vi "odor temporal control panel with logging no AO1 on air and odor1.vi"() -> ()   [LabVIEW 2021]
uses:
  Image Aquisition - Labview/Image Recorder/experiment state global.vi
  <vilib>/DAQmx/write.llb/DAQmx Write (Digital Bool 1Line 1Point).vi
panel:
  in  "direct control of digital lines":bool
  in  "digital controls":T1
  out "flow rates":T2
  out "setpoints":T3={"Air "=1.0, "odor1"=0.0, "odor2"=0.0, "co2"=0.0}
  in  "gradient settings":T4={"air settings"={"enabled"=TRUE, "temporal ramp type"=enum."Square", "period(s)"=1200.0, "high limit"=4.0, "low limit"=4.0, "duty cycle (sq wave)"=50.0, "phase shift (deg)"=0.0, "value to output when disabled"=1.0}, "odor1 settings"={"enabled"=FALSE, "temporal ramp type"=enum."Sine", "period(s)"=120.0, "high limit"=0.0, "low limit"=0.0, "duty cycle (sq wave)"=50.0, "phase shift (deg)"=0.0, "value to output when disabled"=0.0}, "odor2 settings"={"enabled"=FALSE, "temporal ramp type"=enum."Sine", "period(s)"=120.0, "high limit"=0.0, "low limit"=0.0, "duty cycle (sq wave)"=50.0, "phase shift (deg)"=0.0, "value to output when disabled"=0.0}, "co2 settings"={"enabled"=TRUE, "temporal ramp type"=enum."Triangle", "period(s)"=30.0, "high limit"=500.0, "low limit"=0.0, "duty cycle (sq wave)"=50.0, "phase shift (deg)"=-90.0, "value to output when disabled"=0.0}} {"co2 settings"."value to output when disabled" min=0.0; "co2 settings"."low limit" format="%#_6p"; "odor2 settings"."value to output when disabled" max=100.0; "odor2 settings"."low limit" format="%#_6p"; "odor2 settings"."high limit" max=100.0; "odor1 settings"."value to output when disabled" max=100.0; "odor1 settings"."low limit" format="%#_6p"; "odor1 settings"."high limit" max=100.0; "air settings"."value to output when disabled" max=100.0; "air settings"."low limit" format="%#_6p"; "air settings"."high limit" max=100.0}
  in  "Sync Gradient To Image Aquisition":bool
  in  "enable gradient":bool
  in  "restart gradient":bool
  in  "update period (ms)":u32=100
  in  "stop":bool
  out "error out":errorcluster
  # "restarting gradient also enables output"
  # "maximum amplitude is 100"
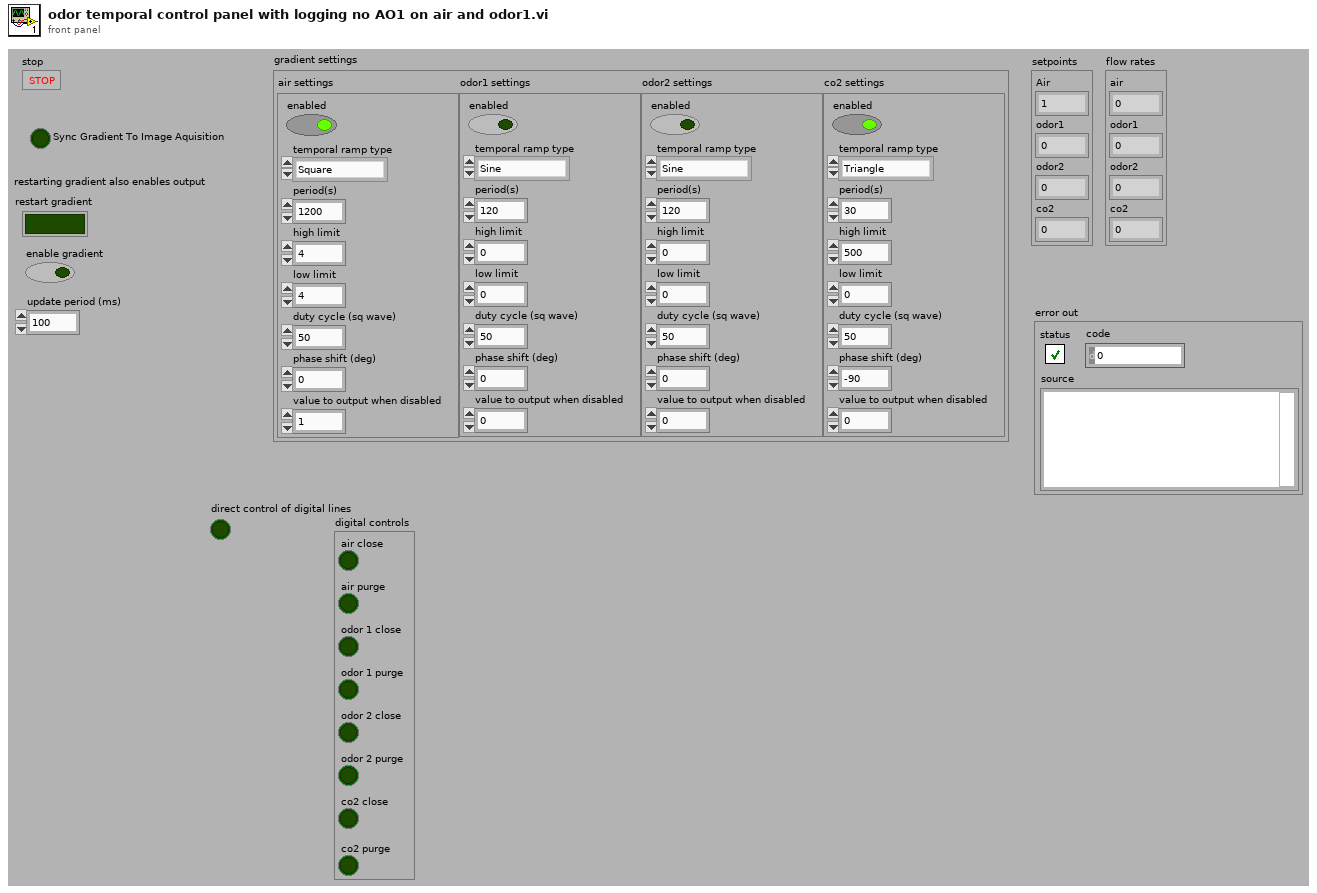
[diagram p1: front panel]
types:
  T1 = cluster{"air close":bool, "air purge":bool, "odor 1 close":bool, "odor 1 purge":bool, "odor 2 close":bool, "odor 2 purge":bool, "co2 close":bool, "co2 purge":bool}
  T2 = cluster{"air":dbl, "odor1":dbl, "odor2":dbl, "co2":dbl}
  T3 = cluster{"Air ":dbl, "odor1":dbl, "odor2":dbl, "co2":dbl}
  T4 = cluster{"air settings":cluster{"enabled":bool, "temporal ramp type":enum16{"Sine", "Triangle", "Sawtooth", "Square", "Exponential"}, "period(s)":dbl, "high limit":dbl, "low limit":dbl, "duty cycle (sq wave)":dbl, "phase shift (deg)":dbl, "value to output when disabled":dbl}, "odor1 settings":cluster{"enabled":bool, "temporal ramp type":enum16{"Sine", "Triangle", "Sawtooth", "Square", "Exponential"}, "period(s)":dbl, "high limit":dbl, "low limit":dbl, "duty cycle (sq wave)":dbl, "phase shift (deg)":dbl, "value to output when disabled":dbl}, "odor2 settings":cluster{"enabled":bool, "temporal ramp type":enum16{"Sine", "Triangle", "Sawtooth", "Square", "Exponential"}, "period(s)":dbl, "high limit":dbl, "low limit":dbl, "duty cycle (sq wave)":dbl, "phase shift (deg)":dbl, "value to output when disabled":dbl}, "co2 settings":cluster{"enabled":bool, "temporal ramp type":enum16{"Sine", "Triangle", "Sawtooth", "Square", "Exponential"}, "period(s)":dbl, "high limit":dbl, "low limit":dbl, "duty cycle (sq wave)":dbl, "phase shift (deg)":dbl, "value to output when disabled":dbl}}
  T5 = cluster{"analog output channels":cluster{"air ao":refnum<k21>, "odor 1 ao":refnum<k21>, "odor 2 ao":refnum<k21>, "co2 ao":refnum<k21>}, "analog input channels":cluster{"air ai":refnum<k21>, "odor 1 ai":refnum<k21>, "odor 2 ai":refnum<k21>, "co2 ai":refnum<k21>, "pid sensor 1 ai":refnum<k21>, "pid sensor 2 ai":refnum<k21>}, "digital control lines":cluster{"air close":refnum<k21>, "air purge":refnum<k21>, "odor 1 close":refnum<k21>, "odor 1 purge":refnum<k21>, "odor 2 close":refnum<k21>, "odor 2 purge":refnum<k21>, "co2 close":refnum<k21>, "co2 purge":refnum<k21>}}
  T6 = cluster{"experiment started":bool, "experiment ended":bool, "experiment start time":u32}
  T7 = cluster{"air close":refnum<k21>, "air purge":refnum<k21>, "odor 1 close":refnum<k21>, "odor 1 purge":refnum<k21>, "odor 2 close":refnum<k21>, "odor 2 purge":refnum<k21>, "co2 close":refnum<k21>, "co2 purge":refnum<k21>}
  T8 = cluster{"air":dbl, "odor1":dbl, "odor2":dbl, "co2":dbl, "pid reading":dbl}
  T9 = cluster{"data directory":path, "file stub":string}
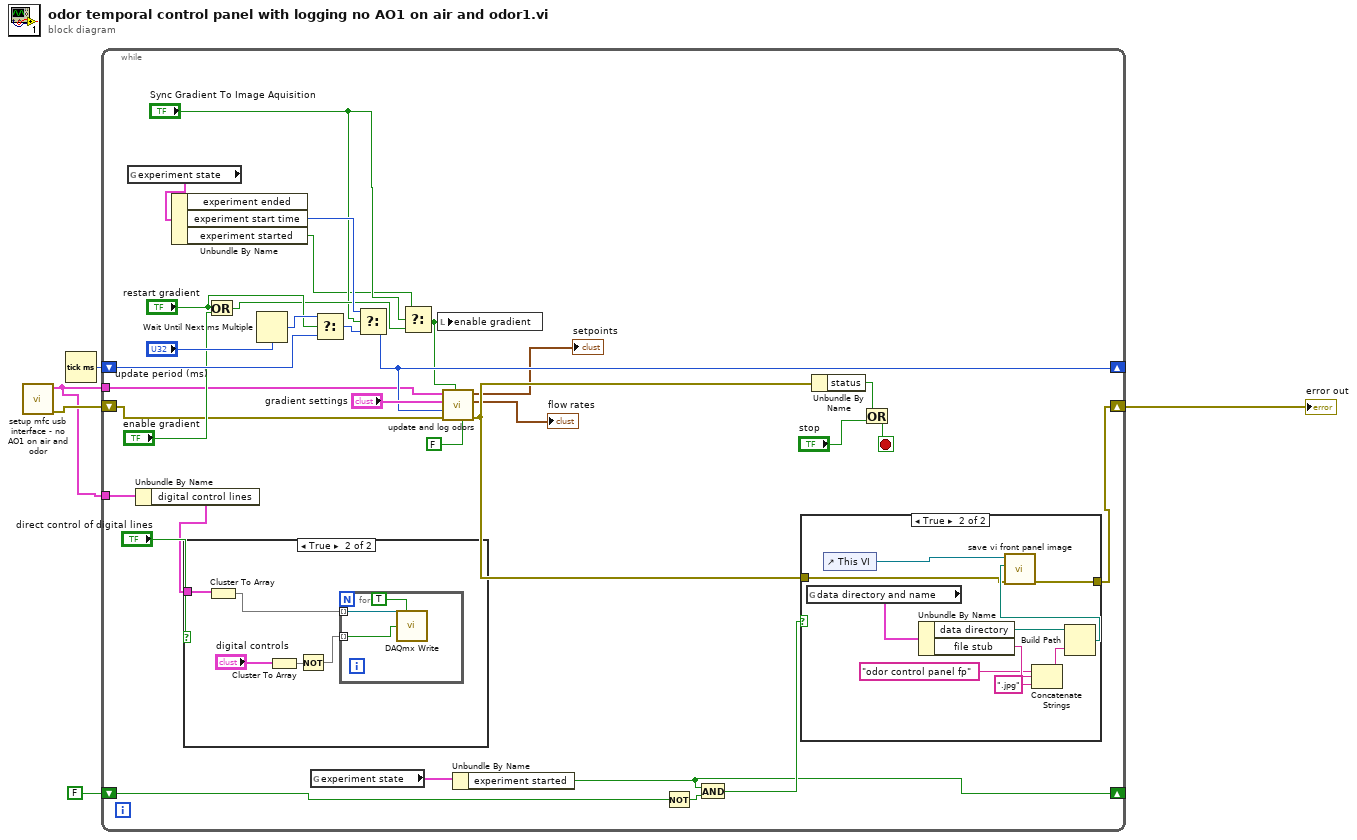
[diagram p0: block diagram]
diagram:
  n1 = call "setup mfc usb interface - no AO1 on air and odor.vi"() -> ("error out"=w4:errorcluster, "daqmx tasks"=w1:T5)  [unwired: 10 in]
  n2 = Tick Count (ms)() -> (millisecond timer value=w5:u32)
  n3 = while {
    shift-right: [w18] -> w3
    shift-left: w4 -> [w15]
    shift-right: [w16] -> _
    shift-left: w5 -> [w34]
    tunnel: w1 -> [w13]
    shift-right: [w20] -> _
    shift-left: FALSE ("experiment started") -> [w19]
    tunnel: w1 -> [w9]
    stop <- w37 stop-if-true
    n4 = global read "experiment state global.vi" "experiment state"() -> (w29:T6)
    n5 = Unbundle By Name(w9) -> ("digital control lines"=w7:T7)
    n6 = Unbundle By Name(w29) -> ("experiment start time"=w28:u32, "experiment started"=w24:bool)  [unwired: 1 out]
    n7 = case shown="True" "direct control of digital lines" {
      tunnel: w7 -> [_ w41]
      frame False {
      }
      frame True {
        n8 = Cluster To Array(cluster=w41) -> (array=w39:refnum<k21>[])
        n9 = Cluster To Array(cluster="digital controls") -> (array=w40:bool[])
        n10 = Not(x=w40) -> (.not. x?=w38:bool[])
        n11 = for {
          tunnel: w39 -> [w45] mode=indexing
          tunnel: w38 -> [w44] mode=indexing
          n12 = call-poly <vilib>:"DAQmx Write.vi"("task/channels in"=w45, "auto start"=TRUE, "data"=w44) -> ()  [unwired: 10 in, 3 out]
        }
      }
    }
    n13 = Or(x="restart gradient", y="enable gradient") -> (x .or. y?=w27:bool)
    n14 = Wait Until Next ms Multiple(millisecond multiple="update period (ms)") -> (millisecond timer value=w33:u32)
    n15 = global read "experiment state global.vi" "experiment state"() -> (w21:T6)
    n16 = Select(t=w33, s="restart gradient", f=w34) -> (s? t:f=w30:u32)
    n17 = Select(t=w28, s="Sync Gradient To Image Aquisition", f=w30) -> (s? t:f=w16:u32)
    n18 = Select(t=w24, s="Sync Gradient To Image Aquisition", f=w27) -> (s? t:f=w14:bool)
    n19 = local write "enable gradient"(w14) -> ()
    n20 = call "update and log odors.vi"("odor 1 enabled?"=FALSE, "global enable"=w14, "error in"=w15, "t0"=w16, "gradient settings"="gradient settings", "daqmx tasks"=w13) -> ("error out"=w12:errorcluster, "flow rates"=→"flow rates":T8, "setpoints"=→"setpoints":T3)  [unwired: 3 in]
    n21 = Unbundle By Name(w21) -> ("experiment started"=w20:bool)
    n22 = Not(x=w19) -> (.not. x?=w23:bool)
    n23 = And(x=w20, y=w23) -> (x .and. y?=w22:bool)
    n24 = case shown="True" w22 {
      tunnel: [w46 w48] -> w18
      tunnel: w12 -> [w46 w47]
      frame False {
      }
      frame True {
        n25 = global read "experiment state global.vi" "data directory and name"() -> (w55:T9)
        n26 = control-ref of="This VI"() -> (w56:refnum<vi>)
        n27 = Unbundle By Name(w55) -> ("data directory"=w54:path, "file stub"=w53:string)
        n28 = Concatenate Strings("odor control panel fp" ("string"), w53, ".jpg" ("string")) -> (w50:string)
        n29 = Build Path(base path=w54, name or relative path=w50) -> (appended path=w49:path)
        n30 = call "save vi front panel image.vi"("error in (no error)"=w47, "path to JPEG file"=w49, "This VI"=w56) -> ("error out"=w48:errorcluster)  [unwired: 8 in]
      }
    }
    n31 = Unbundle By Name(w12) -> ("status"=w31:bool)
    n32 = Or(x=w31, y="stop") -> (x .or. y?=w37:bool)
  }
  "error out" <- w3
